vi "Get Row Indexes Of Unread Errors.vi"(1 "Is Error Read?":bool[](array[boolean])) -> (0 "Row Index Of Unread Errors":i32[](array[numeric]))   [LabVIEW 2023, in "Error Manager.lvlib"]
doc: "This VI returns the row indexes of rows that represent unread errors."
uses:
  Error Manager.lvlib
panel:
  # "Development\nControls or indicators that are useful for development or testing, but which are not outputs of the VI."
  # "Input\nInputs to the VI"
  # "Output\nOutputs of the VI"
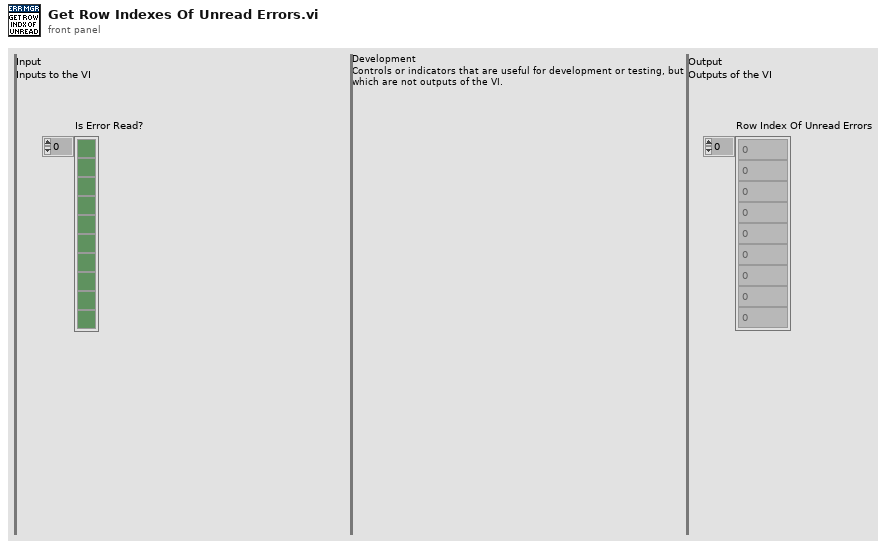
[diagram p1: front panel]
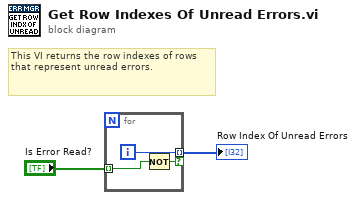
[diagram p0: block diagram]
diagram:
  # "This VI returns the row indexes of rows that represent unread errors."
  n1 = for {
    tunnel: "Is Error Read?" -> [w4] mode=indexing
    tunnel: [w5] -> w1 mode=indexing if=w3
    i -> [w5]
    n2 = Not(x=w4) -> (.not. x?=w3:bool)
  }
  "Row Index Of Unread Errors" <- w1
